vi "AlazarGetSDKVersion.vi"(11 "error in (no error)":errorcluster) -> (4 "Major Number":u8, 6 "Minor Number":u8, 8 "Revision Number":u8, 10 "Return Code":u32, 15 "error out":errorcluster)   [LabVIEW 2018]
doc: "Get the driver library version. This is the version of ATSApi.dll under Windows, or ATSApi.so under Linux."
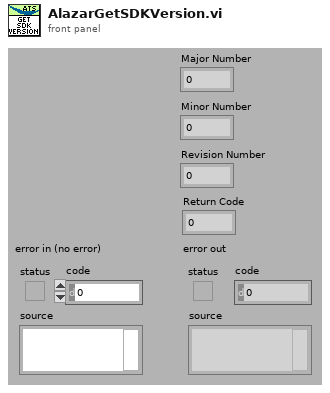
[diagram p1: front panel]
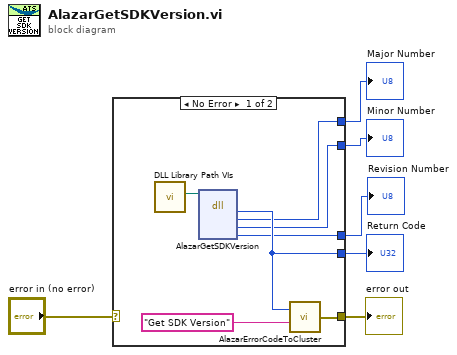
[diagram p0: block diagram]
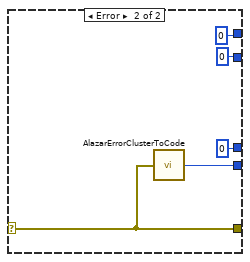
[diagram p2: hidden frame]
diagram:
  n1 = case shown="No Error" "error in (no error)" {
    selector: "error in (no error)" -> [_ w18]
    tunnel: [w11 w18] -> w5
    tunnel: [w13 w17] -> w4
    tunnel: [w10 0] -> w3
    tunnel: [w9 0] -> w2
    tunnel: [w8 0] -> w1
    frame No Error {
      n2 = call "DLL Library Path VIs.vi"() -> ("GPUFFT"=w7:path)  [unwired: 9 in, 2 out]
      n3 = dll-call lib="C:/Project/SerialSectOCT - FFT GPU/SerialSectOCT/Labview Software/DLL/ATSApi.dll" fn="AlazarGetSDKVersion"(path in=w7) -> ("return type"=w13:u32, "majorVersion"=w10:u8, "minorVersion"=w9:u8, "revisionNumber"=w8:u8)  [unwired: 5 in, 2 out]
      n4 = call "AlazarErrorCodeToCluster.vi"("Message"="Get SDK Version", "Error Code"=w13) -> ("error out"=w11:errorcluster)
    }
    frame Error {
      n5 = call "AlazarErrorClusterToCode.vi"("error in (no error)"=w18) -> ("Error Code"=w17:u32)
    }
  }
  "error out" <- w5
  "Return Code" <- w4
  "Major Number" <- w3
  "Minor Number" <- w2
  "Revision Number" <- w1
